vi "QueryHealthAndStatus.vi"(11 "HealthAndStatusSettings":T1={"InternalHealthAndStatusFIFO"="InternalHealthAndStatusFIFO", "HealthAndStatusQueryFIFO"="HealthAndStatusQueryFIFO", "HealthAndStatusResponseFIFO"="HealthAndStatusResponseFIFO", "HealthAndStatusMemory"="HealthAndStatusMemory", "MemorySize"=0}) -> ()   [LabVIEW 2018, in "FPGAHealthAndStatus.lvlib"]
uses:
  FPGAHealthAndStatus.lvlib
  DataTypes/HealthAndStatusSettings.ctl
  DataTypes/QueryHealthAndStatusLoopData.ctl
  DataTypes/QueryHealthAndStatusStates.ctl
  <vilib>/rvi/Emulation/niFpgaGetClockAttributes.vi
  <vilib>/rvi/Emulation/niFpgaSctlEmulationGetInTimedLoop.vi
  <vilib>/rvi/Emulation/niFpgaEmulationReportErrorSimple.vi
  <vilib>/rvi/DataTransferAndStorage/Container/Common/niFpgaContainerExecOnDevCompGetState.vi
  <vilib>/rvi/Emulation/niFpgaEmulationIsFPGAContextNoSignature.vi
  <vilib>/rvi/DataTransferAndStorage/Container/Common/niFpgaContainerGetUniqueNameForEmu.vi
  <vilib>/rvi/Emulation/niFpgaProcessEmulError.vi
  <vilib>/rvi/errors/nirviReportUnexpectedCaseInternalError (U32).vi
  <vilib>/rvi/Memory/Memory_Emulation/niFpgaMemoryEmulationCacheClearOnFirstRun.vi
  <vilib>/rvi/Memory/Memory_Emulation/nirvimemoryEmulationManagerCache_MakeExclusive.vi
  <vilib>/rvi/Memory/Memory_Emulation/niFpgaMemoryEmulationValidateCache.vi
  <vilib>/rvi/Memory/Memory_Emulation/nirvimemoryEmulationManagerCache_InsertValue.vi
  <vilib>/Utility/error.llb/Clear Errors.vi
  <vilib>/rvi/Memory/Memory_Emulation/nirvimemoryEmulationManagerCache_ReleaseExclusive.vi
  <vilib>/rvi/Memory/Memory_Emulation/nirvimemoryEmulationManagerCache_GetValue.vi
  <vilib>/rvi/Memory/Memory_Emulation/nirvimemoryEmulationManagerCache_SetValue.vi
  <vilib>/rvi/Emulation/niFpgaSctlEmulationResourceMgr.vi
  <vilib>/rvi/errors/niFpgaSetErrorForExecOnDevCompSimple.vi
  <vilib>/rvi/eio/common/nirviEmuReportErrorAndStop.vi
  <vilib>/rvi/FIFO/Fifo_Resource/nirvififoEmulationSetSize.vi
  <vilib>/rvi/FIFO/Fifo_Resource/nirviFifoEmulationQueueMgr.vi
  <instcachedir>/0/nirviFifoEmulationQueueMgr_E5CAEC123FF24DC58D834DCA3CDAA9B5.lvgen/nirviFifoEmulationQueueMgr_E5CAEC123FF24DC58D834DCA3CDAA9B5_005.vi
  <vilib>/rvi/FIFO/Fifo_Resource/nirvififoEmulationDetermineInputValidOut.vi
  <vilib>/rvi/FIFO/Fifo_Resource/nirvififoEmulationCreateLock.vi
  <vilib>/rvi/FIFO/Fifo_Resource/nirvififoEmulationObtainLock.vi
  <vilib>/rvi/FIFO/Fifo_Resource/nirvififoEmulationReleaseLock.vi
  <vilib>/rvi/occurrence/nirviWaitOnOccurrenceBase.vi
  <vilib>/rvi/errors/nirviReportUnexpectedCaseInternalError.vi
  <vilib>/rvi/interface/RandomDataEmulation/niFpgaRandomDataHandleErrors.vi
  <vilib>/rvi/Emulation/niFpgaCriticalErrorInLSC.vi
  <vilib>/rvi/DataTransferAndStorage/Container/XNode/niFpgaContainer.xnode
  <vilib>/rvi/Memory/Memory_Emulation/niFpgaMemoryEmulationRefIn.vi
  <vilib>/rvi/FIFO/Fifo_Resource/niFpgaFifoEmulationRefIn.vi
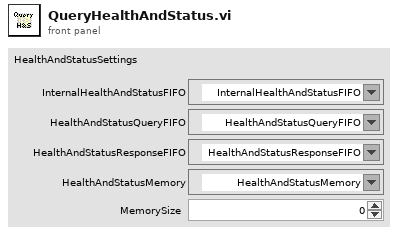
[diagram p1: front panel]
types:
  T1 = typedef "FPGAHealthAndStatus.lvlib/HealthAndStatusSettings.ctl" = cluster{"InternalHealthAndStatusFIFO":refnum<k21>, "HealthAndStatusQueryFIFO":refnum<k21>, "HealthAndStatusResponseFIFO":refnum<k21>, "HealthAndStatusMemory":refnum<k21>, "MemorySize":i32}
  T2 = typedef "FPGAHealthAndStatus.lvlib/QueryHealthAndStatusLoopData.ctl" = cluster{"State":T3, "InstructionData":u64, "AddressOffset":u32}
  T3 = typedef "FPGAHealthAndStatus.lvlib/QueryHealthAndStatusStates.ctl" = enum16{"Try Read Instruction", "Send Telemetry", "Send All Telemetry"}
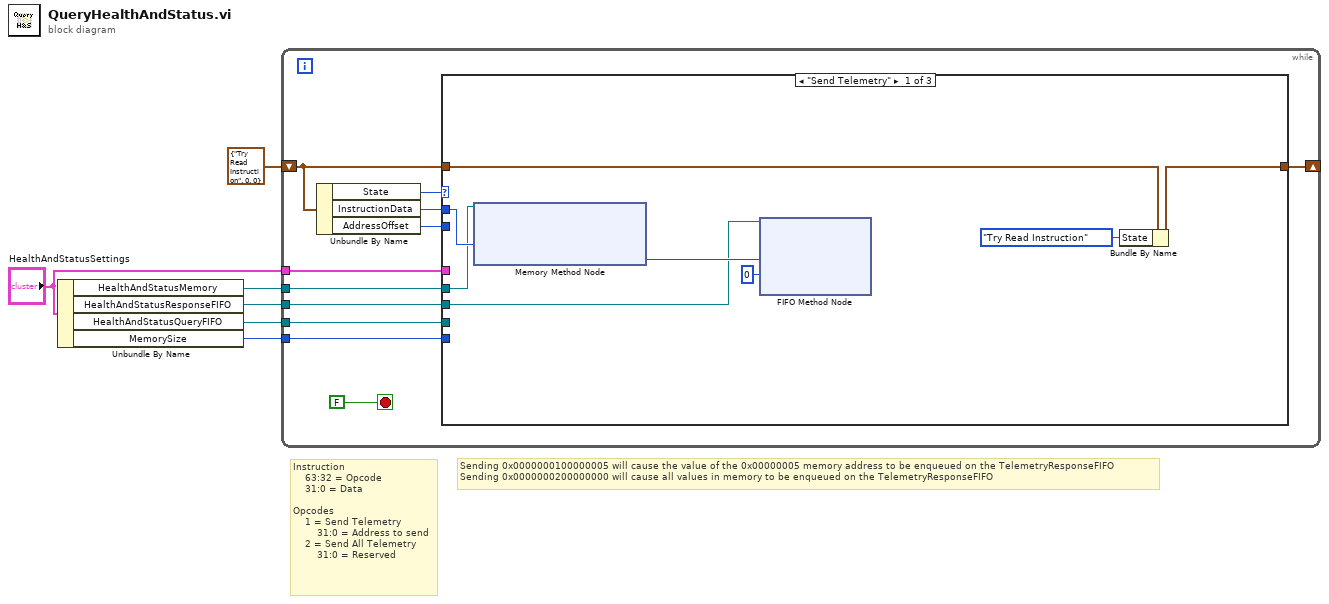
[diagram p0: block diagram]
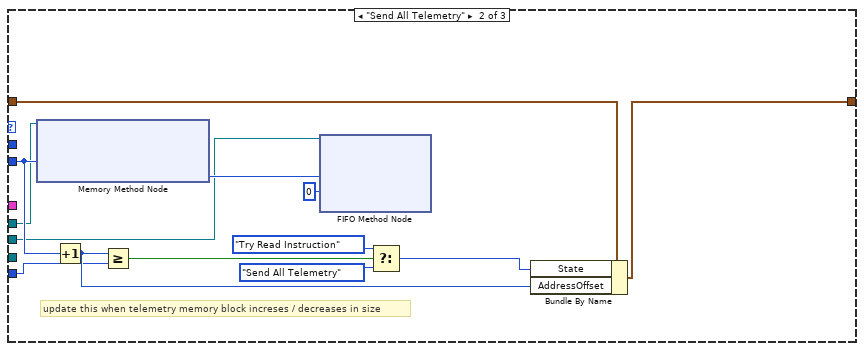
[diagram p2: hidden frame]
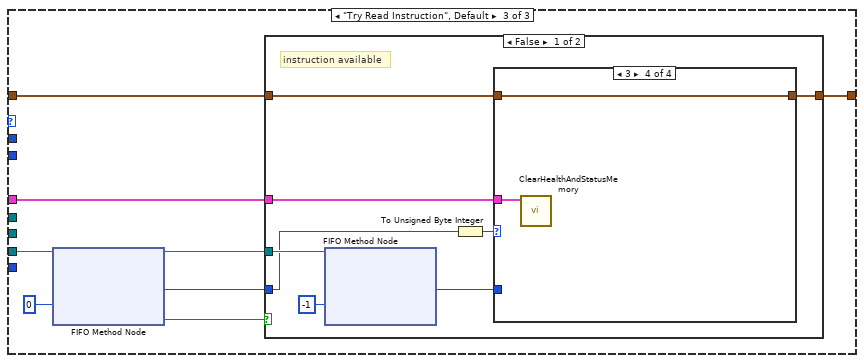
[diagram p3: hidden frame]
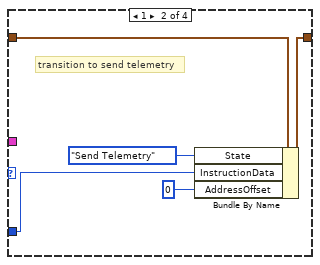
[diagram p5: hidden frame]
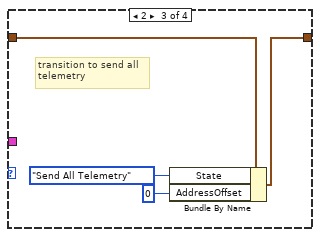
[diagram p6: hidden frame]
diagram:
  # "Sending 0x0000000100000005 will cause the value of the 0x00000005 memory address to be enqueued on the TelemetryResponseFIFO\nSending 0x0000000200000000 will cause all values in memory to be enqueued on the TelemetryResponseFIFO"
  # "Instruction\n    63:32 = Opcode\n    31:0 = Data\n\nOpcodes\n    1 = Send Telemetry\n        31:0 = Address to send\n    2 = Send All Telemetry\n        31:0 = Reserved"
  n1 = Unbundle By Name("HealthAndStatusSettings") -> ("HealthAndStatusMemory"=w2:refnum<k21>, "HealthAndStatusResponseFIFO"=w3:refnum<k21>, "HealthAndStatusQueryFIFO"=w4:refnum<k21>, "MemorySize"=w5:i32)
  n2 = while {
    shift-right: [w14] -> _
    shift-left: T2 {"State"=enum."Try Read Instruction", "InstructionData"=0, "AddressOffset"=0} ("Command Telemetry Loop") -> [w16]
    tunnel: w4 -> [w11]
    tunnel: w2 -> [w10]
    tunnel: w3 -> [w9]
    tunnel: w5 -> [w8]
    tunnel: "HealthAndStatusSettings" -> [w7]
    stop <- FALSE stop-if-true
    n3 = Unbundle By Name(w16) -> ("State"=w17:T3, "InstructionData"=w15:u64, "AddressOffset"=w13:u32)
    n4 = case shown="\"Send Telemetry\"" w17 {
      tunnel: w16 -> [w25 w38 w45]
      tunnel: w15 -> [w23 _ _]
      tunnel: [w24 w37 w44] -> w14
      tunnel: w13 -> [_ w34 _]
      tunnel: w11 -> [_ _ w41]
      tunnel: w10 -> [w19 w28 _]
      tunnel: w9 -> [w18 w27 _]
      tunnel: w8 -> [_ w26 _]
      tunnel: w7 -> [_ _ w40]
      frame "Send Telemetry" {
        n5 = xnode ("Memory Method Node")("Address"=w23, "Memory In"=w19) -> ("Data"=w21:u64)  [unwired: 1 out]
        n6 = xnode ("FIFO Method Node")("Element"=w21, "Timeout"=0, "FIFO In"=w18) -> ()  [unwired: 2 out]
        n7 = Bundle By Name(cluster=w25, "State"=QueryHealthAndStatusStates."Try Read Instruction" ("f")) -> (w24:T2)
      }
      frame "Send All Telemetry" {
        # "update this when telemetry memory block increses / decreases in size"
        n8 = xnode ("Memory Method Node")("Address"=w34, "Memory In"=w28) -> ("Data"=w36:u64)  [unwired: 1 out]
        n9 = Increment(x=w34) -> (x+1=w29:u32)
        n10 = Greater Or Equal?(x=w29, y=w26) -> (x >= y?=w33:bool)
        n11 = xnode ("FIFO Method Node")("Element"=w36, "Timeout"=0, "FIFO In"=w27) -> ()  [unwired: 2 out]
        n12 = Select(t=QueryHealthAndStatusStates."Try Read Instruction" ("f"), s=w33, f=QueryHealthAndStatusStates."Send All Telemetry") -> (s? t:f=w30:T3)
        n13 = Bundle By Name(cluster=w38, "State"=w30, "AddressOffset"=w29) -> (w37:T2)
      }
      frame "Try Read Instruction", Default {
        n14 = xnode ("FIFO Method Node")("Timeout"=0, "FIFO In"=w41) -> ("Element"=w46:u64, "Timed Out?"=w42:bool, "FIFO Out"=w39:refnum<k21>)
        n15 = case shown="False" w42 {
          tunnel: w46 -> [w47 _]
          tunnel: w45 -> [w54 w67]
          tunnel: [w53 w67] -> w44
          tunnel: w40 -> [w52 _]
          tunnel: w39 -> [w51 _]
          frame False {
            # "instruction available"
            n16 = xnode ("FIFO Method Node")("Timeout"=-1, "FIFO In"=w51) -> ("Element"=w49:u64)  [unwired: 2 out]
            n17 = To Unsigned Byte Integer(number=w47) -> (unsigned 8bit integer=w48:u8)
            n18 = case shown="3" w48 {
              tunnel: w54 -> [w55 w60 w64 w66]
              tunnel: [w55 w59 w63 w66] -> w53
              tunnel: w49 -> [_ w56 _ _]
              tunnel: w52 -> [_ _ _ w65]
              frame 0, Default {
                # "nop"
              }
              frame 1 {
                # "transition to send telemetry"
                n19 = Bundle By Name(cluster=w60, "State"=QueryHealthAndStatusStates."Send Telemetry", "InstructionData"=w56, "AddressOffset"=u32 0 ("Telemetry Offset")) -> (w59:T2)
              }
              frame 2 {
                # "transition to send all \ntelemetry"
                n20 = Bundle By Name(cluster=w64, "State"=QueryHealthAndStatusStates."Send All Telemetry", "AddressOffset"=u32 0 ("Telemetry Offset")) -> (w63:T2)
              }
              frame 3 {
                n21 = call "ClearHealthAndStatusMemory.vi"("HealthAndStatusSettings"=w65) -> ()  [unwired: 11 in]
              }
            }
          }
          frame True {
            # "no instruction available"
          }
        }
      }
    }
  }
